vi "DAQ External Sampling.vi"() -> ()   [LabVIEW 2013]
uses:
  <vilib>/DAQmx/read.llb/DAQmx Read (Analog 1D DBL 1Chan NSamp).vi
  <vilib>/DAQmx/create/channels.llb/DAQmx Create Channel (AI-Voltage-Basic).vi
  <vilib>/DAQmx/configure/timing.llb/DAQmx Timing (Sample Clock).vi
  <vilib>/DAQmx/miscellaneous.llb/DAQmx Fill In Error Info.vi
panel:
  out "Waveform Chart":dbl[](graph)
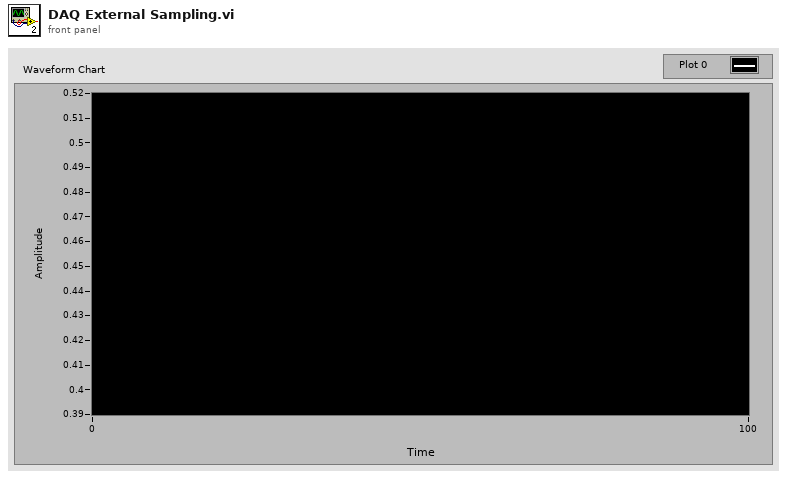
[diagram p1: front panel]
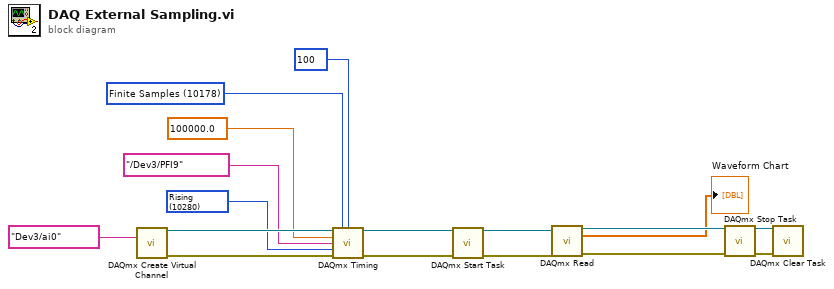
[diagram p0: block diagram]
diagram:
  w11 = 10178 items=["Finite Samples"=10178, "Continuous Samples"=10123, "Hardware Timed Single Point"=12522] ("sample mode")
  w14 = 10280 items=["Rising"=10280, "Falling"=10171] ("active edge")
  n1 = call-poly <vilib>:"DAQmx Create Virtual Channel.vi"("physical channels"=tag "Dev3/ai0") -> ("task out"=w16:refnum<k21>, "error out"=w15:errorcluster)  [unwired: 13 in]
  n2 = call-poly <vilib>:"DAQmx Timing.vi"("task/channels in"=w16, "sample mode"=w11, "samples per channel"=100, "rate"=100000.0, "source"=tag "/Dev3/PFI9", "active edge"=w14, "error in"=w15) -> ("task out"=w1:refnum<k21>, "error out"=w9:errorcluster)  [unwired: 7 in]
  n3 = call <vilib>:"DAQmx Start Task.vi"("task/channels in"=w1, "error in"=w9) -> ("task out"=w8:refnum<k21>, "error out"=w7:errorcluster)  [unwired: 12 in]
  n4 = call-poly <vilib>:"DAQmx Read.vi"("task/channels in"=w8, "error in"=w7) -> ("task out"=w6:refnum<k21>, "data"=→"Waveform Chart":dbl[], "error out"=w5:errorcluster)  [unwired: 11 in]
  n5 = call <vilib>:"DAQmx Stop Task.vi"("task/channels in"=w6, "error in"=w5) -> ("task out"=w4:refnum<k21>, "error out"=w3:errorcluster)  [unwired: 12 in]
  n6 = call <vilib>:"DAQmx Clear Task.vi"("task in"=w4, "error in"=w3) -> ()  [unwired: 13 in, 1 out]
